vi "read_registers_ASIC.vi"() -> ()   [LabVIEW 2009]
panel:
  in  "Data":i32
  out "data out serial":string
  out "Array 2":T1(array[cluster])
  out "Array":T2(array[cluster])
  in  "array of registers to read":i32[](array[numeric])=[0, 1, 2, 3, 4, 10, 11, 12, 13, 14, 15, 16, 23, 24, 25, 26, 27, 28, 29, 30, 31]
  in  "Id in":u32
  out "total cycles":i32
  out "bucle":i32
  out "data read value":u32
  out "error out 2":errorcluster
  in  "error in (no error)":errorcluster
  out "Id in":u32
  in  "Read physical":bool=TRUE
  out "Data to send hex":string
  in  "Device":u16(ring)=4 items=["Attenuation", "Clipping", "Enable channel", "Delay line", "ASIC"]
  in  "Read/#write":bool
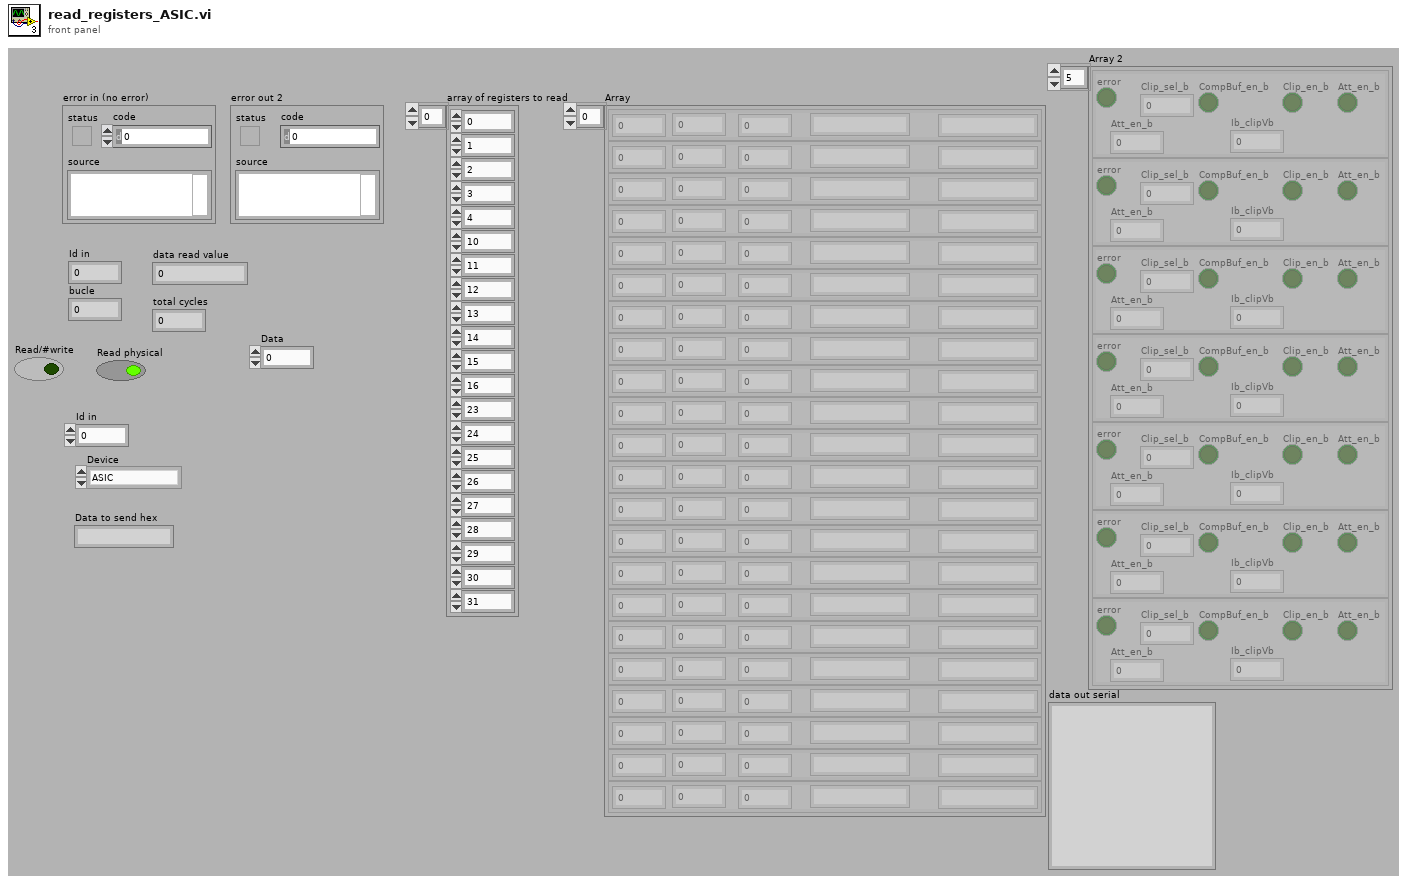
[diagram p1: front panel]
types:
  T1 = cluster{"error":bool, "Clip_sel_b":u32, "Att_en_b":u32, "CompBuf_en_b":bool, "Clip_en_b":bool, "Att_en_b":bool, "Ib_clipVb":u32}[]
  T2 = cluster{u32, i32, u32, "data out serial":string, "hex integer string":string}[]
  T3 = cluster{u32, i32, u32, "data out serial":string, "hex integer string":string}
  T4 = cluster{"error":bool, "Clip_sel_b":u32, "Att_en_b":u32, "CompBuf_en_b":bool, "Clip_en_b":bool, "Att_en_b":bool, "Ib_clipVb":u32}
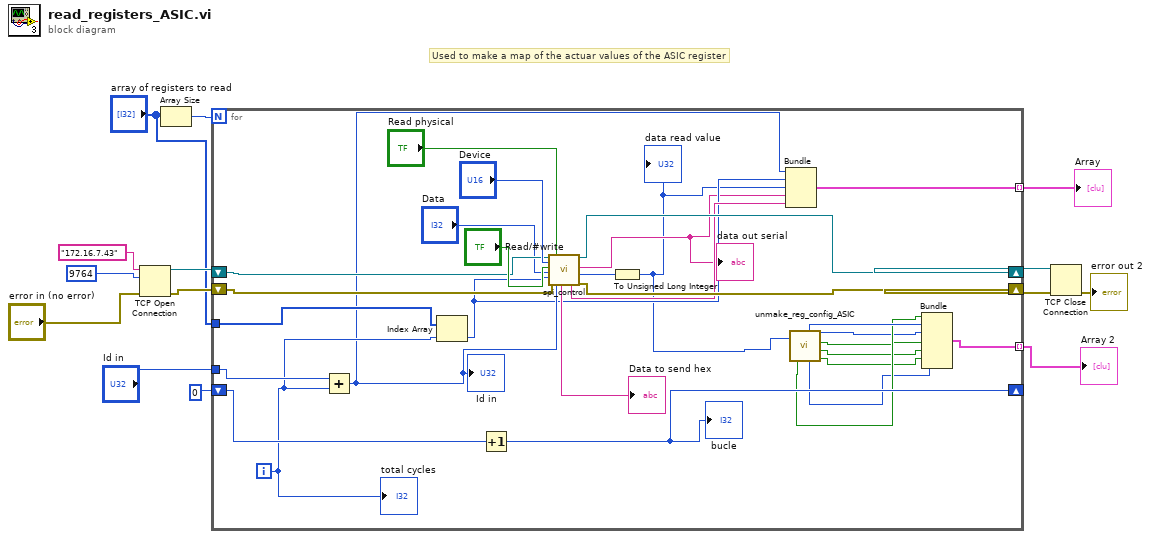
[diagram p0: block diagram]
diagram:
  # "Used to make a map of the actuar values of the ASIC register"
  n1 = TCP Open Connection(address="172.16.7.43", remote port or service name=u16 9764, error in (no error)="error in (no error)") -> (connection ID=w10:refnum<k5>, error out=w9:errorcluster)  [unwired: 2 in]
  n2 = Array Size(array="array of registers to read") -> (size(s)=w3:i32)
  n3 = for {
    N: w3 -> [_]
    shift-right: [w43] -> w12
    shift-left: w9 -> [w34]
    shift-right: [w42] -> w11
    shift-left: w10 -> [w33]
    shift-right: [w40] -> _
    shift-left: 0 ("lower limit") -> [w41]
    tunnel: "Id in" -> [w32]
    tunnel: "array of registers to read" -> [w30]
    tunnel: [w25] -> w2 mode=indexing
    tunnel: [w16] -> w1 mode=indexing
    i -> [w31]
    n4 = Add(x=w32, y=w31) -> (x+y=w29:u32)
    "Id in" <- w29
    n5 = Index Array(array=w30, index=w31) -> (element=w27:i32)
    n6 = Increment(x=w41) -> (x+1=w40:i32)
    "bucle" <- w40
    n7 = call "spi_control.vi"("connection ID"=w33, "Device"="Device", "Read/#write"="Read/#write", "Data"="Data", "Register or channel"=w27, "error out 3"=w34, "Read physical"="Read physical", "Id in"=w29) -> ("Data to send hex"=→"Data to send hex":string, "hex integer string"=w28:string, "connection ID out"=w42:refnum<k5>, "data out serial"=w26:string, "data read value"=w35:u32, "error out 2"=w43:errorcluster)  [unwired: 4 in, 2 out]
    "data out serial" <- w26
    n8 = To Unsigned Long Integer(number=w35) -> (unsigned 32bit integer=w24:u32)
    "data read value" <- w24
    n9 = Bundle(w29, w27, w24, "data out serial"=w26, "hex integer string"=w28) -> (w25:T3)  [unwired: 1 in]
    n10 = call "unmake_reg_config_ASIC.vi"("In_reg_value"=w24) -> ("error"=w22:bool, "Clip_sel_b"=w23:u32, "Ib_clipVb"=w17:u32, 4:"Att_en_b"=w21:u32, "CompBuf_en_b"=w20:bool, "Clip_en_b"=w19:bool, 7:"Att_en_b"=w18:bool)
    n11 = Bundle("error"=w22, "Clip_sel_b"=w23, "Att_en_b"=w21, "CompBuf_en_b"=w20, "Clip_en_b"=w19, "Att_en_b"=w18, "Ib_clipVb"=w17) -> (w16:T4)  [unwired: 1 in]
    "total cycles" <- w31
  }
  "Array" <- w2
  "Array 2" <- w1
  n12 = TCP Close Connection(connection ID=w11, error in (no error)=w12) -> (error out=→"error out 2":errorcluster)  [unwired: 1 in, 1 out]
